vi "Microscope Control.vi"() -> ()   [LabVIEW 2016]
uses:
  Tabs.ctl
panel:
  in  "Stop":bool
  in  "Menu":bool
  in  "MenuCluster":T1
  out "Tab Control":T2
  in  "Access/Refresh Token Path":path
  in  "BMP MAIN FOLDER":path
  in  "Create Page":bool
  in  "Send Image To Onenote?":bool
  out "2D Picture":picture
  out "Current_Inkscape Path":path
  in  "Open_InkScape_dialogue":bool
  # "This will be for all of the settings behind the scenes that the user should not see."
  # "Images"
  # "OneNote"
  # "OneNote Tab"
  # "I should have a control that will let me open the lithography program (this should be done via the command line)."
  # "I wanna show the lithography process as it is happening."
  # "I should get a confirmation that the image is saved and I should also see if I cant display it here."
  # "I think that I want to make a full blown VI that will do literally everything.\nThat means I need to plan out the structure of the VI before I start. I would \nlike to make things like a hamburger menu and a a thing that displays the \ncorrect front panel of whatever im doing etc. In other words I wanna make a boss ass program for the microscope."
  # "The border and label should get hidden."
  # "I should hide the tabs, make this transparent, and then programmatically change the tabs."
  # "Experiment with adding states to the beginning and end of the  queue to change the states a little more  readily..."
  # "ALL NOTES SHOULD GO HERE"
  # "Colors:\nMicroscope: rgb(238,105,66) or near this color\nOnenote:  R128 G57 B123\nPaths: path color (blueish green)\ninkscape"
  # "This  is the Default tab"
  # "The way I shall organize this large undertaking:\nI will make a series of Sub VIs. \nThe main app reference will be in the main VI\nAll references should be opened and closed inside of the sub VIs\nThis will ensure that we will not have any lose hanging references.\nI will also have a series of onenote cases."
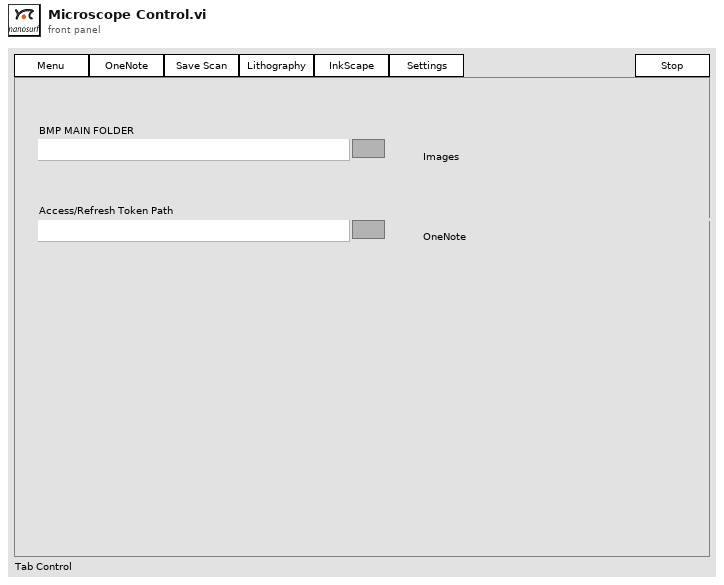
[diagram p1: front panel]
types:
  T1 = cluster{"Settings":bool, "Save Scan":bool, "Perform Lithography":bool, "Open InkScape":bool, "Onenotebutton":bool}
  T2 = typedef "Tabs.ctl" = enum32{"Settings", "Onenote", "Lithography", "Save Image", "InkScape", "Default"}
  T3 = enum32{"invalid app kind", "Development System", "Run Time System", "Student Edition", "Embedded LabVIEW", "Evaluation", "Custom"}
  T4 = enum32{"Invalid", "Standard", "Closed", "Hidden", "Minimized", "Maximized"}
  T5 = cluster{"Core":cluster{"Current VI Reference":refnum<vi>, "Close Panel on Exit?":bool}, "Your Boolean data":bool, "Your string data":string, "Application":refnum<k7>, "Paths":cluster{"BMP_Str":string, "BMP_INK_Str":string, "InkScape_Str":string, "BMP_path":path, "BMP_INK_Path":path, "InkScape_Path":path, "BasePath":path}, "Scan Properties":cluster{"CenterPosX":dbl, "CenterPosY":dbl, "ImageHeight":dbl, "ImageWidth":dbl}, "OneNote":cluster{"Description":string, "Body":cluster{"Description":string, "Path":path}[]}}
  T6 = cluster{"Description":string, "Body":cluster{"Description":string, "Path":path}[]}
  T7 = cluster{"CenterPosX":dbl, "CenterPosY":dbl, "ImageHeight":dbl, "ImageWidth":dbl}
  T8 = cluster{"BMP_Str":string, "BMP_INK_Str":string, "InkScape_Str":string, "BMP_path":path, "BMP_INK_Path":path, "InkScape_Path":path, "BasePath":path}
  T9 = cluster{"Current VI Reference":refnum<vi>, "Close Panel on Exit?":bool}
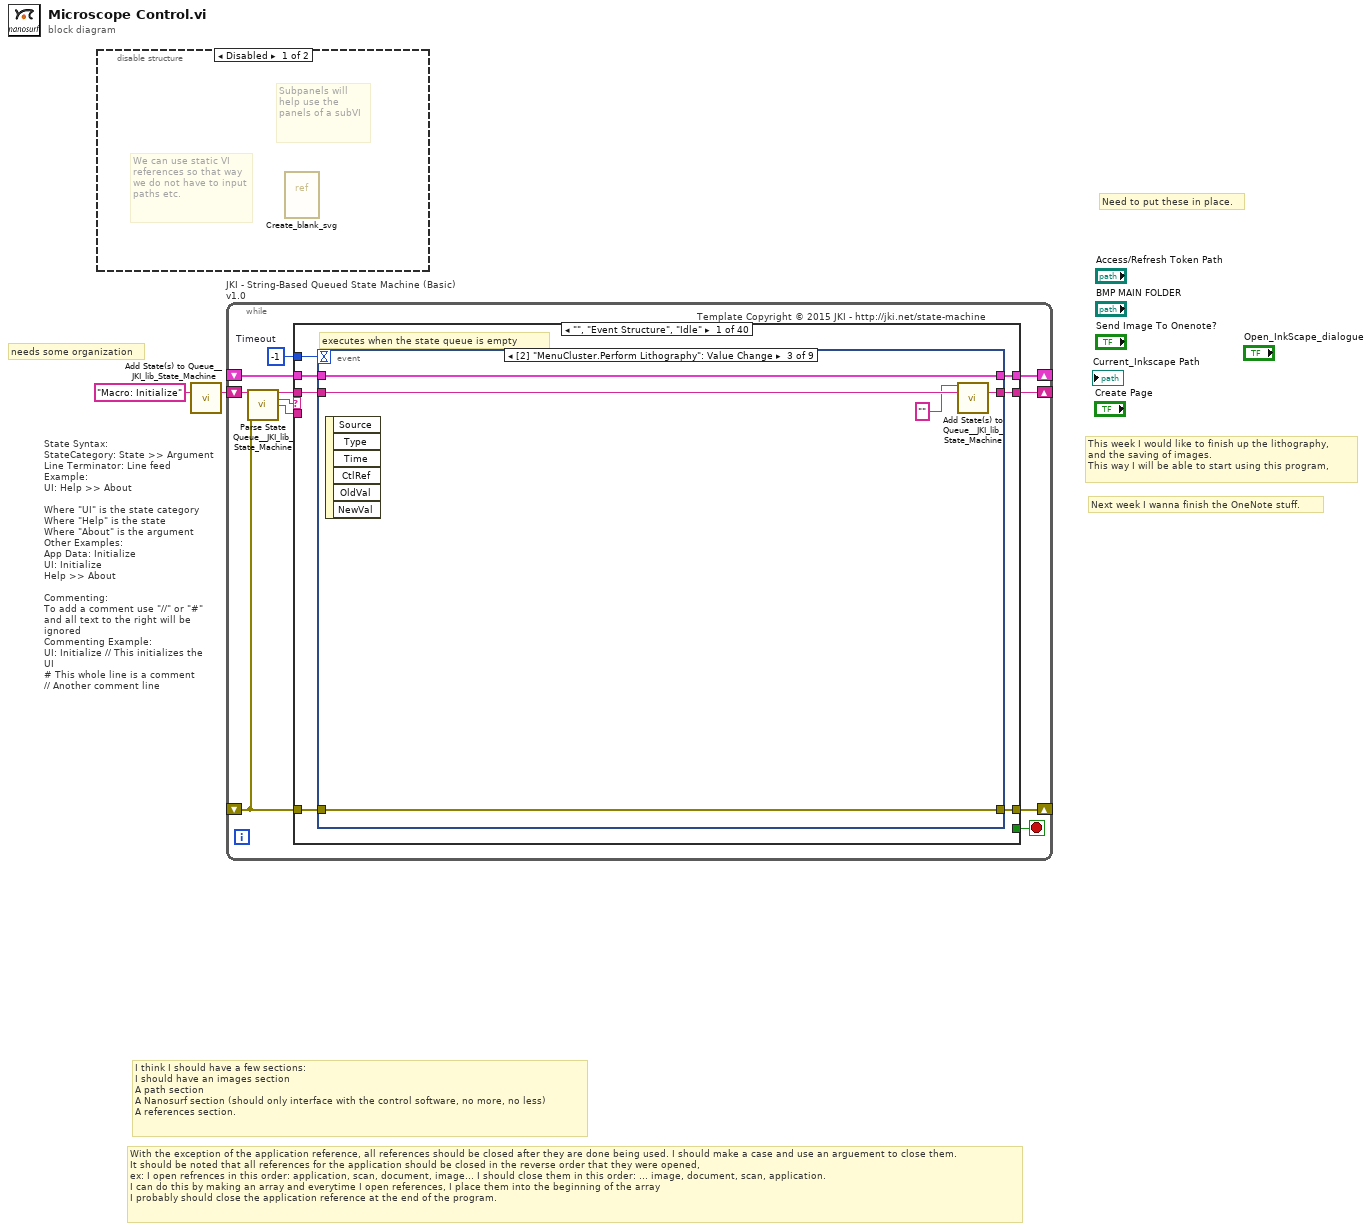
[diagram p0: block diagram]
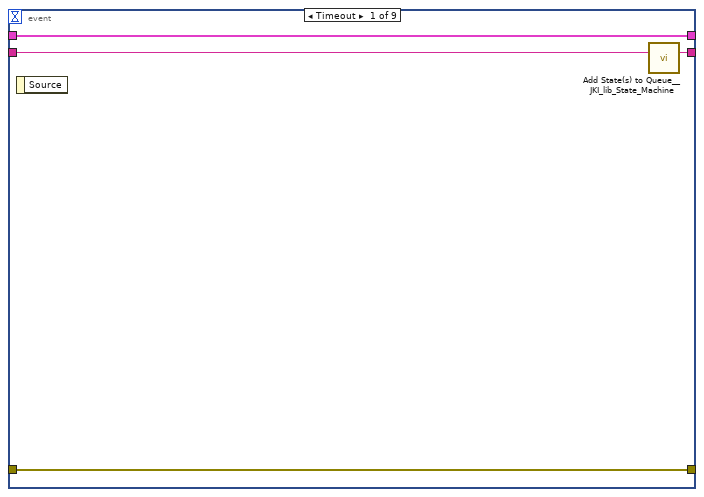
[diagram p3: hidden frame]
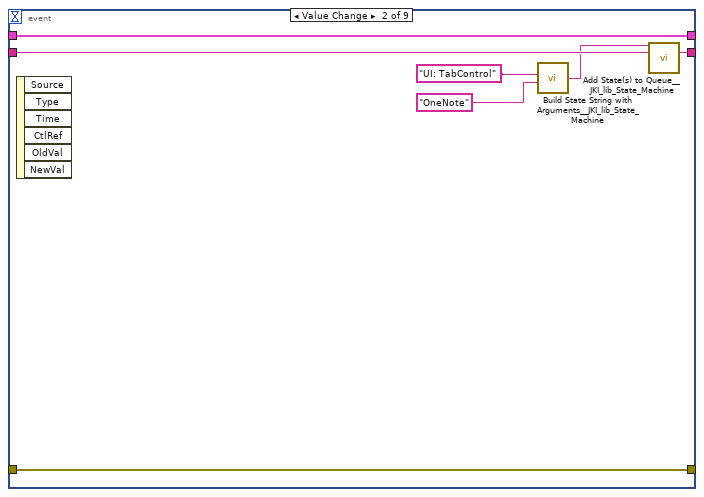
[diagram p4: hidden frame]
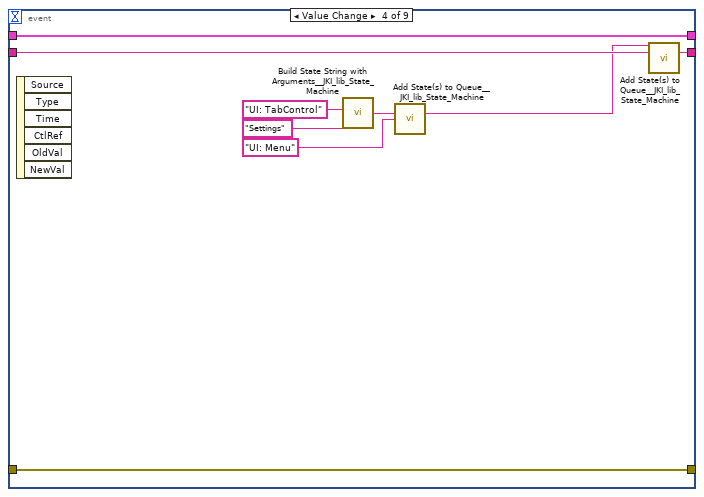
[diagram p5: hidden frame]
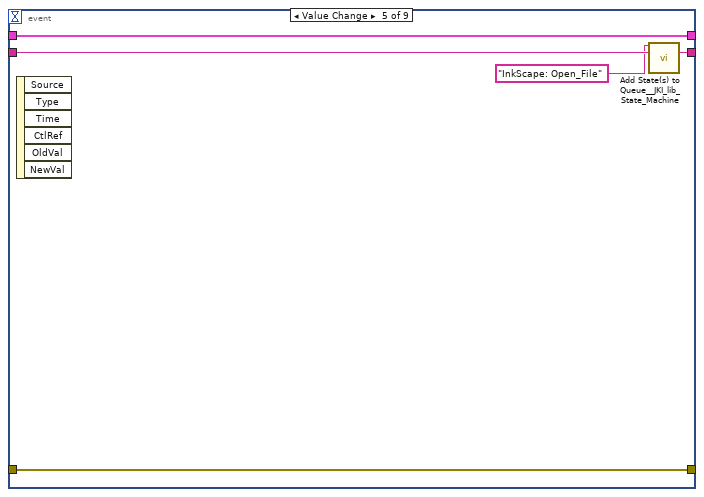
[diagram p6: hidden frame]
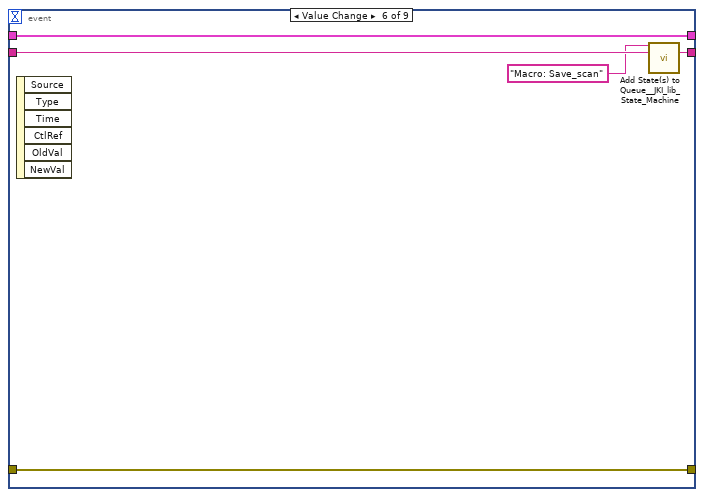
[diagram p7: hidden frame]
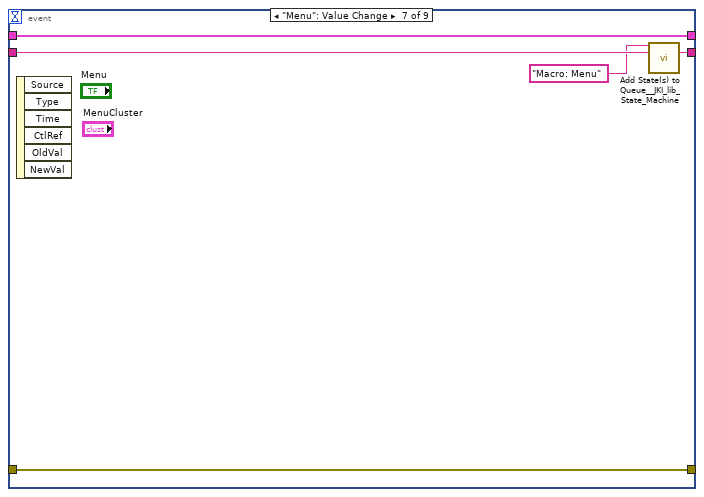
[diagram p8: hidden frame]
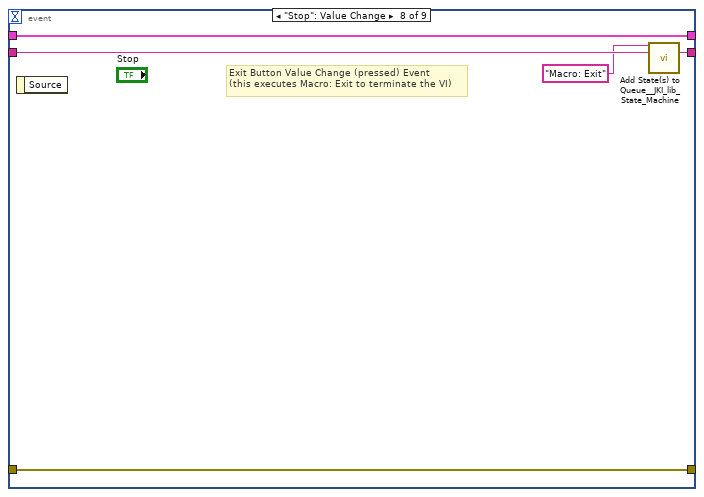
[diagram p9: hidden frame]
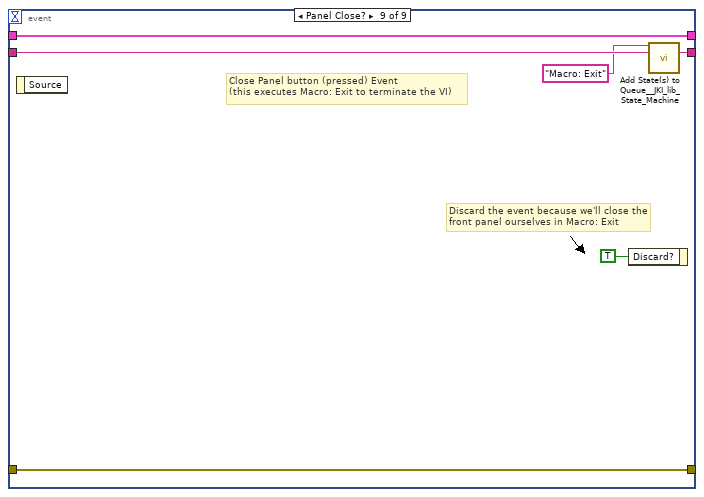
[diagram p10: hidden frame]
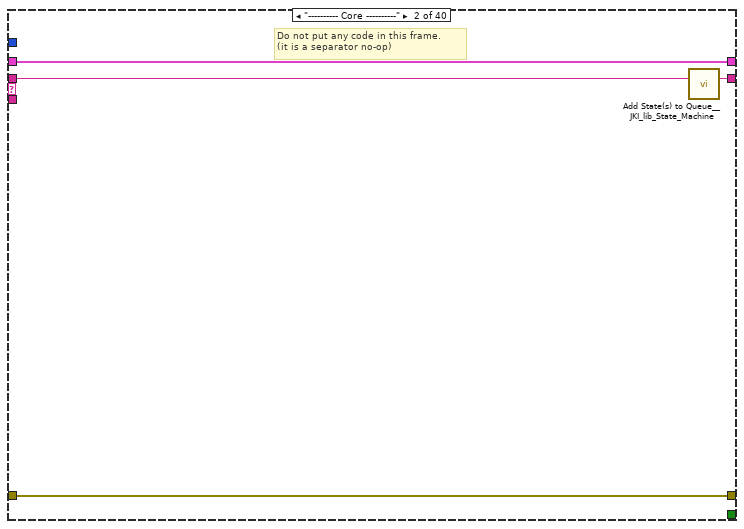
[diagram p11: hidden frame]
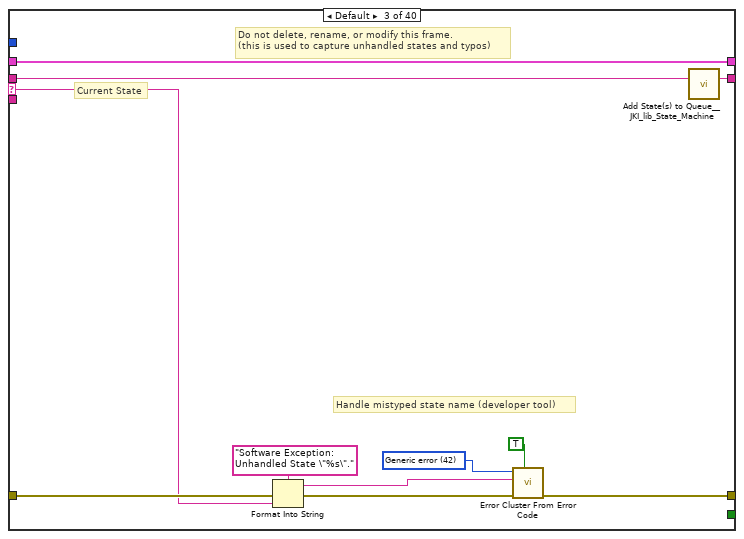
[diagram p12: hidden frame]
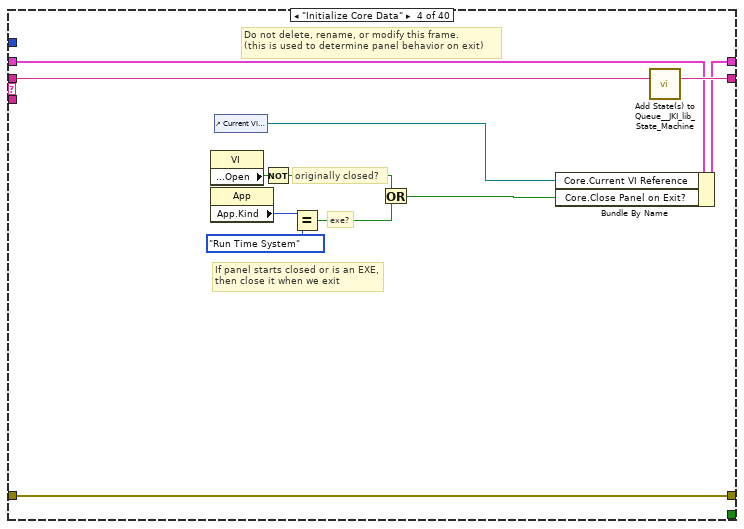
[diagram p13: hidden frame]
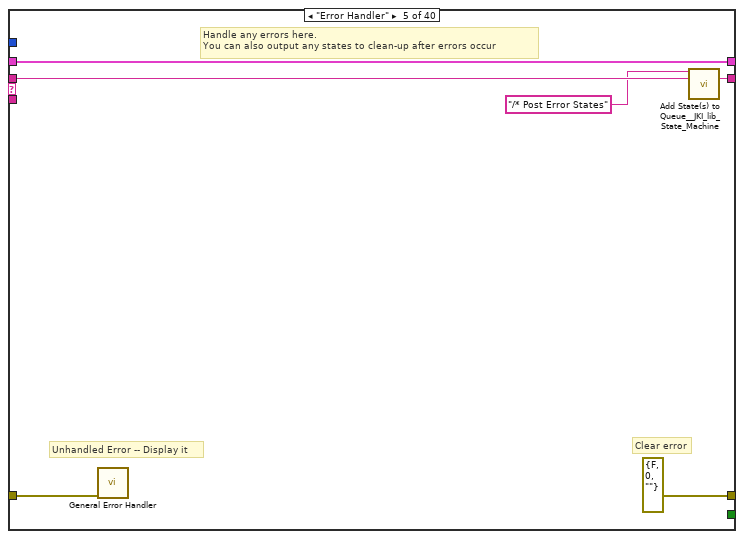
[diagram p14: hidden frame]
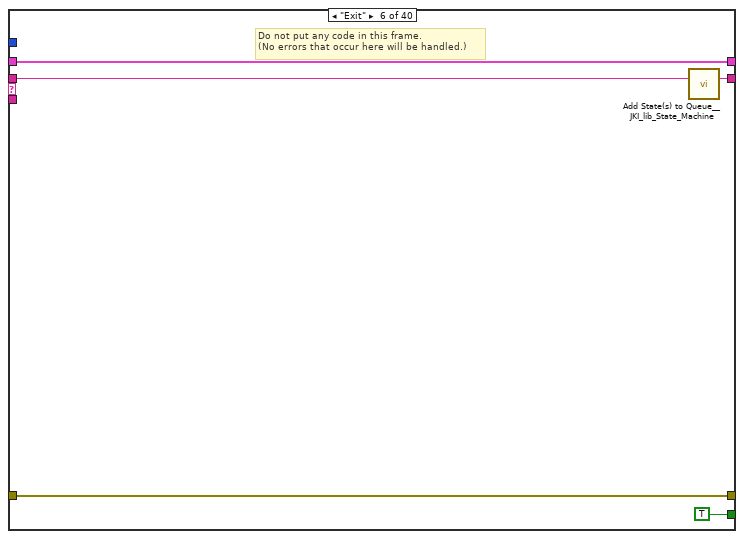
[diagram p15: hidden frame]
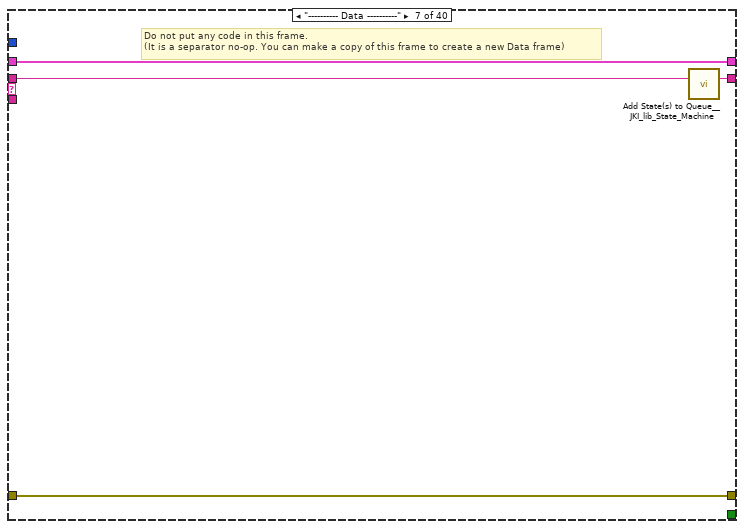
[diagram p16: hidden frame]
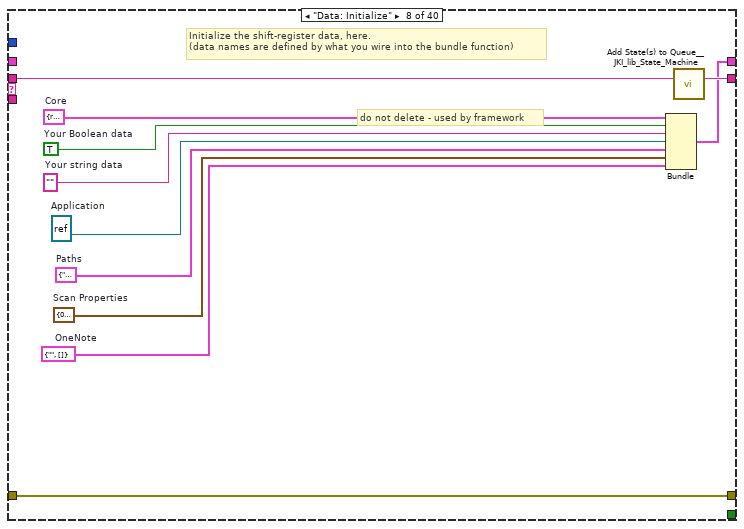
[diagram p17: hidden frame]
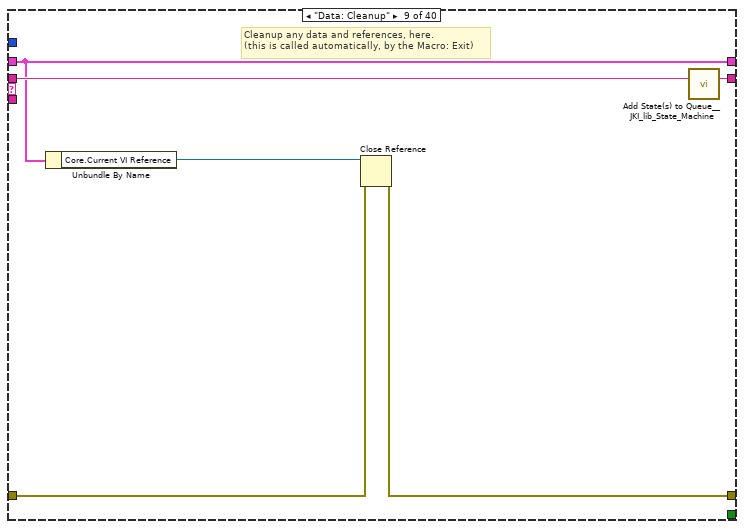
[diagram p18: hidden frame]
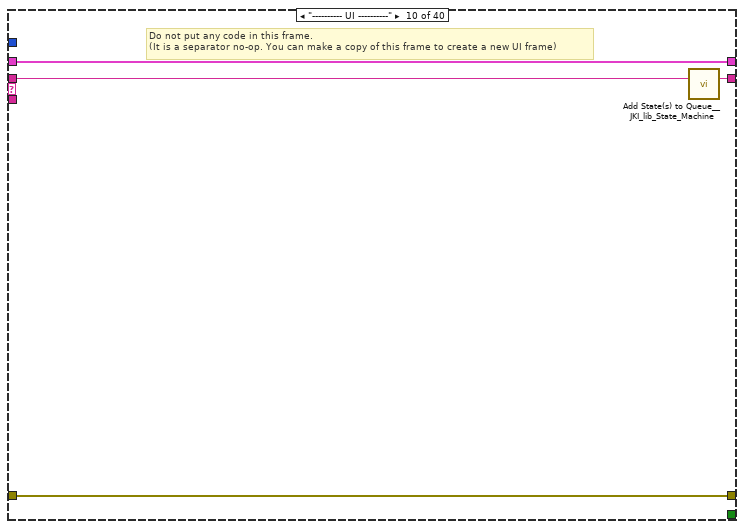
[diagram p19: hidden frame]
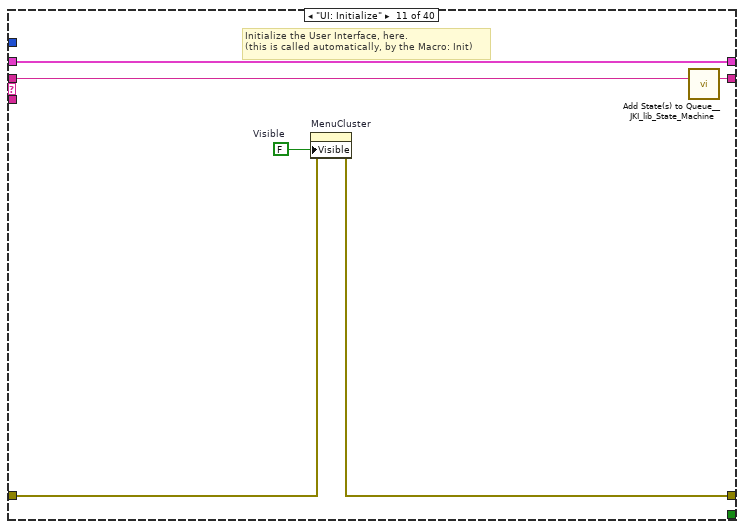
[diagram p20: hidden frame]
diagram:
  # "Need to put these in place."
  # "Next week I wanna finish the OneNote stuff."
  # "This week I would like to finish up the lithography, \nand the saving of images. \nThis way I will be able to start using this program,"
  # "With the exception of the application reference, all references should be closed after they are done being used. I should make a case and use an arguement to close them.\nIt should be noted that all references for the application should be closed in the reverse order that they were opened,\nex: I open refrences in this order: application, scan, document, image... I should close them in this order: ... image, document, scan, application.\nI can do this by making an array and everytime I open references, I place them into the beginning of the array\nI probably should close the application reference at the end of the program."
  # "I think I should have a few sections:\nI should have an images section\nA path section\nA Nanosurf section (should only interface with the control software, no more, no less)\nA references section."
  # "needs some organization"
  # "State Syntax:\nStateCategory: State >> Argument\nLine Terminator: Line feed\nExample:\nUI: Help >> About\n\nWhere \"UI\" is the state category\nWhere \"Help\" is the state\nWhere \"About\" is the argument\nOther Examples:\nApp Data: Initialize\nUI: Initialize\nHelp >> About\n\nCommenting:\nTo add a comment use \"//\" or \"#\" and all text to the right will be ignored\nCommenting Example:\nUI: Initialize // This initializes the UI\n# This whole line is a comment\n// Another comment line"
  n1 = disable-structure shown="Disabled" {
    frame Disabled {
      # "Subpanels will help use the panels of a subVI"
      # "We can use static VI references so that way we do not have to input paths etc."
      n2 = vi-ref "Create_blank_svg.vi"() -> ()  [unwired: 1 out]
    }
    frame Enabled {
    }
  }
  n3 = call <vilib>:"Add State(s) to Queue__JKI_lib_State_Machine.vi"("State(s) in (\"\")"="Macro: Initialize") -> ("States Out"=w2:string)  [unwired: 14 in]
  n4 = while "JKI - String-Based Queued State Machine (Basic) v1.0" {
    shift-right: [w6] -> _
    shift-left: _ -> [w5]
    shift-right: [w9] -> _
    shift-left: _ -> [w3]
    shift-right: [w8] -> _
    shift-left: w2 -> [w10]
    stop <- w7 stop-if-true
    w4 = -1  # Timeout
    # "Template Copyright © 2015 JKI - http://jki.net/state-machine"
    n5 = call <vilib>:"Parse State Queue__JKI_lib_State_Machine.vi"("State Queue"=w10, "Error In (no error)"=w3) -> ("Remaining States"=w12:string, "Current State"=w13:string, "Arguments"=w11:string)  [unwired: 11 in]
    n6 = case shown="\"\", \"Event Structure\", \"Idle\"" w13 {
      selector: w13 -> [_ _ w76 _ _ _ _ _ _ _ _ _ _ _ _ _ _ _ _ _ _ _ _ _ _ _ _ _ _ _ _ _ _ _ _ _ _ _ _ _]
      tunnel: w12 -> [w20 w75 w80 w98 w104 w109 w113 w124 w130 w134 w140 w146 w157 w187 w193 w202 w207 w212 w217 w222 w231 w244 w253 w266 w270 w278 w292 w304 w310 w314 w321 w327 w331 w342 w353 w357 w362 w373 w378 w384]
      tunnel: w11 -> [_ _ _ _ _ _ _ _ _ _ _ w141 w151 _ w188 _ _ _ _ _ _ _ _ _ _ _ _ _ _ _ _ _ _ _ _ _ _ _ _ _]
      tunnel: w5 -> [w18 w72 w78 w89 w101 w107 w110 _ w125 w131 w138 w144 w153 w185 w190 w199 w204 w209 w214 w219 w229 w241 w250 w262 w267 w273 w290 w295 w308 w311 w319 w325 w328 w336 w345 w354 w360 w364 w376 w380]
      tunnel: [w17 w73 w82 w95 errorcluster {"status"=FALSE, "code"=0, "source"=""} ("error out") w106 w111 w121 w126 w132 w135 w142 w154 w180 w191 w200 w205 w210 w215 w220 w227 w242 w251 w263 w268 w275 w280 w302 w305 w312 w315 w322 w329 w339 w346 w355 w358 w371 w374 w381] -> w9
      tunnel: w3 -> [w16 w73 w81 w95 w100 w106 w111 w121 w127 w132 w136 w143 w155 w181 w191 w200 w205 w210 w215 w220 w228 w242 w251 w254 w268 w271 w287 w293 w306 w312 w316 w323 w329 w340 w347 w355 w359 w371 w375 w382]
      tunnel: [w19 w74 w79 w97 w103 w108 w112 w123 w129 w133 w139 w145 w156 w186 w192 w201 w206 w211 w216 w221 w230 w243 w252 w265 w269 w277 w291 w303 w309 w313 w320 w326 w330 w341 w352 w356 w361 w372 w377 w383] -> w8
      tunnel: [_ _ _ _ _ TRUE _ _ _ _ _ _ _ _ _ _ _ _ _ _ _ _ _ _ _ _ _ _ _ _ _ _ _ _ _ _ _ _ _ _] -> w7
      tunnel: [w15 w72 w78 w96 w101 w107 w110 w122 w125 w131 w138 w144 w153 w185 w190 w199 w204 w209 w214 w219 w229 w241 w250 w261 w267 w276 w290 w294 w308 w311 w319 w325 w328 w335 w345 w354 w360 w363 w376 w380] -> w6
      tunnel: w4 -> [w14 _ _ _ _ _ _ _ _ _ _ _ _ _ _ _ _ _ _ _ _ _ _ _ _ _ _ _ _ _ _ _ _ _ _ _ _ _ _ _]
      frame "", "Event Structure", "Idle" {
        # "executes when the state queue is empty"
        n7 = event shown="[2] \"MenuCluster.Perform Lithography\": Value Change" {
          selector: _ -> [_ _ _ _ _ _ _ _ _]
          dyn-events: _ -> [_ _ _ _ _ _ _ _ _]
          timeout: w14 -> [_ _ _ _ _ _ _ _ _]
          tunnel: w20 -> [w24 w31 w36 w45 w50 w55 w60 w65 w71]
          tunnel: [w23 w30 w35 w44 w49 w54 w59 w64 w70] -> w19
          tunnel: w18 -> [w21 w28 w33 w42 w47 w52 w57 w62 w68]
          tunnel: [w22 w29 w34 w43 w48 w53 w58 w63 w69] -> w17
          tunnel: w16 -> [w22 w29 w34 w43 w48 w53 w58 w63 w69]
          tunnel: [w21 w28 w33 w42 w47 w52 w57 w62 w68] -> w15
          event Timeout {
            n8 = event-data() -> ()  [unwired: 1 in, 1 out]
            n9 = call <vilib>:"Add State(s) to Queue__JKI_lib_State_Machine.vi"("State(s) in (\"\")"=w24) -> ("States Out"=w23:string)  [unwired: 14 in]
          }
          event "MenuCluster.Onenotebutton": Value Change {
            n10 = event-data() -> ()  [unwired: 1 in, 6 out]
            n11 = call <vilib>:"Build State String with Arguments__JKI_lib_State_Machine.vi"("Arguments (\"\")"="OneNote" ("Arguments (\"\")"), "State"="UI: TabControl") -> ("State with Arguments"=w26:string)  [unwired: 4 in]
            n12 = call <vilib>:"Add State(s) to Queue__JKI_lib_State_Machine.vi"("State(s) in Front (\"\")"=w26, "State(s) in (\"\")"=w31) -> ("States Out"=w30:string)  [unwired: 13 in]
          }
          event "MenuCluster.Perform Lithography": Value Change {
            n13 = event-data() -> ()  [unwired: 1 in, 6 out]
            n14 = call <vilib>:"Add State(s) to Queue__JKI_lib_State_Machine.vi"("State(s) in Front (\"\")"="" ("State(s) in Front (\"\")"), "State(s) in (\"\")"=w36) -> ("States Out"=w35:string)  [unwired: 13 in]
          }
          event "MenuCluster.Settings": Value Change {
            n15 = event-data() -> ()  [unwired: 1 in, 6 out]
            n16 = call <vilib>:"Build State String with Arguments__JKI_lib_State_Machine.vi"("Arguments (\"\")"="Settings" ("Arguments (\"\")"), "State"="UI: TabControl") -> ("State with Arguments"=w39:string)  [unwired: 4 in]
            n17 = call <vilib>:"Add State(s) to Queue__JKI_lib_State_Machine.vi"("State(s) in (\"\")"=w39, "State(s) at Back (\"\")"="UI: Menu") -> ("States Out"=w37:string)  [unwired: 13 in]
            n18 = call <vilib>:"Add State(s) to Queue__JKI_lib_State_Machine.vi"("State(s) in Front (\"\")"=w37, "State(s) in (\"\")"=w45) -> ("States Out"=w44:string)  [unwired: 13 in]
          }
          event "MenuCluster.Open InkScape": Value Change {
            n19 = event-data() -> ()  [unwired: 1 in, 6 out]
            n20 = call <vilib>:"Add State(s) to Queue__JKI_lib_State_Machine.vi"("State(s) in Front (\"\")"="InkScape: Open_File", "State(s) in (\"\")"=w50) -> ("States Out"=w49:string)  [unwired: 13 in]
          }
          event "MenuCluster.Save Scan": Value Change {
            n21 = event-data() -> ()  [unwired: 1 in, 6 out]
            n22 = call <vilib>:"Add State(s) to Queue__JKI_lib_State_Machine.vi"("State(s) in Front (\"\")"="Macro: Save_scan" ("State(s) in Front (\"\")"), "State(s) in (\"\")"=w55) -> ("States Out"=w54:string)  [unwired: 13 in]
          }
          event "Menu": Value Change {
            n23 = event-data() -> ()  [unwired: 1 in, 6 out]
            n24 = call <vilib>:"Add State(s) to Queue__JKI_lib_State_Machine.vi"("State(s) in Front (\"\")"="Macro: Menu" ("State(s) in Front (\"\")"), "State(s) in (\"\")"=w60) -> ("States Out"=w59:string)  [unwired: 13 in]
          }
          event "Stop": Value Change {
            # "Exit Button Value Change (pressed) Event\n(this executes Macro: Exit to terminate the VI)"
            n25 = event-data() -> ()  [unwired: 1 in, 1 out]
            n26 = call <vilib>:"Add State(s) to Queue__JKI_lib_State_Machine.vi"("State(s) in Front (\"\")"="Macro: Exit", "State(s) in (\"\")"=w65) -> ("States Out"=w64:string)  [unwired: 13 in]
          }
          event Panel Close? {
            # "Discard the event because we'll close the front panel ourselves in Macro: Exit"
            # "Close Panel button (pressed) Event\n(this executes Macro: Exit to terminate the VI)"
            n27 = event-data() -> ()  [unwired: 1 in, 1 out]
            n28 = event-data("Discard?"=TRUE) -> ()  [unwired: 1 in, 1 out]
            n29 = call <vilib>:"Add State(s) to Queue__JKI_lib_State_Machine.vi"("State(s) in Front (\"\")"="Macro: Exit", "State(s) in (\"\")"=w71) -> ("States Out"=w70:string)  [unwired: 13 in]
          }
        }
      }
      frame "---------- Core ----------" {
        # "Do not put any code in this frame.\n(it is a separator no-op)"
        n30 = call <vilib>:"Add State(s) to Queue__JKI_lib_State_Machine.vi"("State(s) in (\"\")"=w75) -> ("States Out"=w74:string)  [unwired: 14 in]
      }
      frame Default {
        w85 = 42 items=["No error", "Argument error", "Memory is full", "Out of zone", "End of file", "File already open", "Generic file I/O error", "File not found", "File permission error", "Disk is full", "Duplicate path", "Too many files open", "System feature not enabled", "Resource file not found", "Cannot add resource", "Resource not found", "Image not found", "Image memory error", "Pen does not exist", "Config type invalid", "Config token not found", "Config parse error", "Config memory error", "Bad external code format", "Bad external code offset", "External code not present", "Null window", "Destroy window error", "Null menu", "Print aborted", "Bad print record", "Print driver error", "Windows error during printing", "Memory error during printing", "Print dialog error", "Generic print error", "Invalid device refnum", "Device not found", "Device parameter error", "Device unit error", "Cannot open device", "Device call aborted", "Generic error", "Cancelled by user", "Object ID too low", "Object ID too high", "Object not in heap", "Unknown heap", "Unknown object (invalid DefProc)", "Unknown object (DefProc not in table)", "Message out of range", "Invalid (null) method", "Unknown message", "Manager call not supported", "Bad address", "Network operation in progress", "Network operation timed out", "Connection is busy", "Network attribute not supported", "Network error", "Address in use", "System out of memory", "Connection aborted", "Connection refused", "Not connected", "Already connected", "Connection closed", "Initialization error (interapplication manager)", "Bad occurrence", "Wait on unbound occurrence handler", "Occurrence queue overflow", "Datalog type conflict", "Unused", "Unrecognized type (interapplication manager)", "Memory corrupt", "Failed to make temporary DLL", "Old CIN version", "Drag socket not found", "Failed to load drop-object", "Failed to register OLE object", "Failed to release OLE object", "Format specifier type mismatch", "Unknown format specifier", "Too few format specifiers", "Too many format specifiers", "Scan failed", "Newer CIN version", "Error converting to variant", "Runtime menu error", "Password tampered", "Variant attribute not found", "Incompatible variant data type", "Event data is not available", "Event Store is not present", "Occurrence is not found", "Event Queue is not created", "Event info is not available", "Refnum passed is NULL", "Error retrieving Class GUID", "Error retrieving CoClass GUID", "Error retrieving TypeLib GUID.", "Bad built application magic bytes.", "Specific driver is different from the specific driver associated with the Logical Name.", "There is no session opened to the class driver.", "Max Error", "MAX - Error with config objects", "MAX - Error loading configuration", "MAX - Group not supported"]
        # "Current State"
        # "Do not delete, rename, or modify this frame.\n(this is used to capture unhandled states and typos)"
        # "Handle mistyped state name (developer tool)"
        n31 = Format Into String(format string="Software Exception: Unhandled State \"%s\"." ("message"), error in=w81, w76) -> (resulting string=w84:string, error out=w83:errorcluster)  [unwired: 1 in]
        n32 = call <vilib>:"Error Cluster From Error Code.vi"("show call chain? (False)"=TRUE, "error in (no error)"=w83, "error message (\"\")"=w84, "error code (0)"=w85) -> ("error out"=w82:errorcluster)  [unwired: 5 in]
        n33 = call <vilib>:"Add State(s) to Queue__JKI_lib_State_Machine.vi"("State(s) in (\"\")"=w80) -> ("States Out"=w79:string)  [unwired: 14 in]
      }
      frame "Initialize Core Data" {
        # "Do not delete, rename, or modify this frame.\n(this is used to determine panel behavior on exit)"
        # "originally closed?"
        # "exe?"
        # "If panel starts closed or is an EXE, then close it when we exit"
        n34 = property class="VI"() -> ("Front Panel.Open"=w94:bool)  [unwired: 2 in, 2 out]
        n35 = property class="App"() -> ("App.Kind"=w93:T3)  [unwired: 2 in, 2 out]
        n36 = control-ref of="Current VI Reference"() -> (w87:refnum<vi>)
        n37 = Not(x=w94) -> (.not. x?=w91:bool)
        n38 = Equal?(x=w93, y=T3."Run Time System" ("Application:Kind")) -> (x = y?=w90:bool)
        n39 = Or(x=w91, y=w90) -> (x .or. y?=w88:bool)
        n40 = Bundle By Name(cluster=w89, "Core.Current VI Reference"=w87, "Core.Close Panel on Exit?"=w88) -> (w96:T5)
        n41 = call <vilib>:"Add State(s) to Queue__JKI_lib_State_Machine.vi"("State(s) in (\"\")"=w98) -> ("States Out"=w97:string)  [unwired: 14 in]
      }
      frame "Error Handler" {
        # "Unhandled Error -- Display it"
        # "Handle any errors here.\nYou can also output any states to clean-up after errors occur"
        # "Clear error"
        n42 = call <vilib>:"General Error Handler.vi"("error in (no error)"=w100) -> ()  [unwired: 10 in, 5 out]
        n43 = call <vilib>:"Add State(s) to Queue__JKI_lib_State_Machine.vi"("State(s) in Front (\"\")"="/* Post Error States", "State(s) in (\"\")"=w104) -> ("States Out"=w103:string)  [unwired: 13 in]
      }
      frame "Exit" {
        # "Do not put any code in this frame.\n(No errors that occur here will be handled.)"
        n44 = call <vilib>:"Add State(s) to Queue__JKI_lib_State_Machine.vi"("State(s) in (\"\")"=w109) -> ("States Out"=w108:string)  [unwired: 14 in]
      }
      frame "---------- Data ----------" {
        # "Do not put any code in this frame.\n(It is a separator no-op. You can make a copy of this frame to create a new Data frame)"
        n45 = call <vilib>:"Add State(s) to Queue__JKI_lib_State_Machine.vi"("State(s) in (\"\")"=w113) -> ("States Out"=w112:string)  [unwired: 14 in]
      }
      frame "Data: Initialize" {
        w114 = T6 {"Description"="", "Body"=[]}  # OneNote
        w115 = T7 {"CenterPosX"=0.0, "CenterPosY"=0.0, "ImageHeight"=0.0, "ImageWidth"=0.0}  # Scan Properties
        w116 = T8 {"BMP_Str"="", "BMP_INK_Str"="", "InkScape_Str"="", "BMP_path"=path "", "BMP_INK_Path"=path "", "InkScape_Path"=path "", "BasePath"=path "C:/Users/monke/Desktop"}  # Paths
        w117 = refnum<k7> refnum  # Application
        w118 = T9 {"Current VI Reference"=refnum, "Close Panel on Exit?"=FALSE}  # Core
        w120 = TRUE  # Your Boolean data
        w119 = ""  # Your string data
        # "do not delete - used by framework"
        # "Initialize the shift-register data, here.\n(data names are defined by what you wire into the bundle function)"
        n46 = Bundle("Core"=w118, "Your Boolean data"=w120, "Your string data"=w119, "Application"=w117, "Paths"=w116, "Scan Properties"=w115, "OneNote"=w114) -> (w122:T5)  [unwired: 1 in]
        n47 = call <vilib>:"Add State(s) to Queue__JKI_lib_State_Machine.vi"("State(s) in (\"\")"=w124) -> ("States Out"=w123:string)  [unwired: 14 in]
      }
      frame "Data: Cleanup" {
        # "Cleanup any data and references, here.\n(this is called automatically, by the Macro: Exit)"
        n48 = Unbundle By Name(w125) -> ("Core.Current VI Reference"=w128:refnum<vi>)
        n49 = Close Reference(reference=w128, error in (no error)=w127) -> (error out=w126:errorcluster)
        n50 = call <vilib>:"Add State(s) to Queue__JKI_lib_State_Machine.vi"("State(s) in (\"\")"=w130) -> ("States Out"=w129:string)  [unwired: 14 in]
      }
      frame "---------- UI ----------" {
        # "Do not put any code in this frame.\n(It is a separator no-op. You can make a copy of this frame to create a new UI frame)"
        n51 = call <vilib>:"Add State(s) to Queue__JKI_lib_State_Machine.vi"("State(s) in (\"\")"=w134) -> ("States Out"=w133:string)  [unwired: 14 in]
      }
      frame "UI: Initialize" {
        w137 = FALSE  # Visible
        # "Initialize the User Interface, here.\n(this is called automatically, by the Macro: Init)"
        n52 = property on="MenuCluster" class="Clust"(error in=w136, "Visible"=w137) -> (error out=w135:errorcluster)  [unwired: 1 in, 1 out]
        n53 = call <vilib>:"Add State(s) to Queue__JKI_lib_State_Machine.vi"("State(s) in (\"\")"=w140) -> ("States Out"=w139:string)  [unwired: 14 in]
      }
      frame "UI: Cursor Set" {
        # "Argument"
        # "Set and Unset Cursor Busy.\n(Usage: \"UI: Cursor Set >> Busy|Idle\")"
        n54 = case shown="\"Idle\", Default" w141 {
          tunnel: w143 -> [w148 w150]
          tunnel: [w147 w149] -> w142
          frame "Idle", Default {
            n55 = call <vilib>:"Unset Busy.vi"("error in (no error)"=w148) -> ("error out"=w147:errorcluster)  [unwired: 10 in]
          }
          frame "Busy" {
            n56 = call <vilib>:"Set Busy.vi"("error in (no error)"=w150) -> ("error out"=w149:errorcluster)  [unwired: 9 in, 1 out]
          }
        }
        n57 = call <vilib>:"Add State(s) to Queue__JKI_lib_State_Machine.vi"("State(s) in (\"\")"=w146) -> ("States Out"=w145:string)  [unwired: 14 in]
      }
      frame "UI: Front Panel State" {
        # "Argument"
        # "Set Front Panel Open or Closed\n(Usage: \"UI: Front Panel State >> Open|Close\")"
        n58 = Unbundle By Name(w153) -> ("Core.Current VI Reference"=w152:refnum<vi>)
        n59 = case shown="\"Open\", Default" w151 {
          tunnel: w155 -> [w161 w174]
          tunnel: [w163 w175] -> w154
          tunnel: w152 -> [w162 w172]
          frame "Open", Default {
            n60 = property class="VI"(reference=w162, error in=w161) -> (reference out=w159:refnum<vi>, error out=w160:errorcluster, "Front Panel.Open"=w158:bool)
            n61 = case shown="False" w158 {
              tunnel: [w166 w169] -> w163
              tunnel: w160 -> [w165 w169]
              tunnel: w159 -> [w164 _]
              frame False {
                n62 = invoke class="VI" method="FP.Open"(reference=w164, error in=w165, "Activate"=TRUE, "State"=T4."Standard") -> (error out=w166:errorcluster)  [unwired: 1 in, 4 out]
              }
              frame True {
              }
            }
          }
          frame "Close" {
            n63 = property class="VI"(reference=w172, error in=w174) -> (reference out=w171:refnum<vi>, error out=w173:errorcluster, "Front Panel.Open"=w170:bool)
            n64 = case shown="True" w170 {
              tunnel: [w176 w179] -> w175
              tunnel: w173 -> [w176 w178]
              tunnel: w171 -> [_ w177]
              frame False {
              }
              frame True {
                n65 = invoke class="VI" method="FP.Close"(reference=w177, error in=w178) -> (error out=w179:errorcluster)  [unwired: 1 in, 2 out]
              }
            }
          }
        }
        n66 = call <vilib>:"Add State(s) to Queue__JKI_lib_State_Machine.vi"("State(s) in (\"\")"=w157) -> ("States Out"=w156:string)  [unwired: 14 in]
      }
      frame "UI: Menu" {
        # "Do not put any code in this frame.\n(It is a separator no-op. You can make a copy of this frame to create a new UI frame)"
        n67 = property on="MenuCluster" class="Clust"(error in=w181) -> (error out=w182:errorcluster, "Visible"=w184:bool)  [unwired: 1 in, 1 out]
        n68 = Not(x=w184) -> (.not. x?=w183:bool)
        n69 = property on="MenuCluster" class="Clust"(error in=w182, "Visible"=w183) -> (error out=w180:errorcluster)  [unwired: 1 in, 1 out]
        n70 = call <vilib>:"Add State(s) to Queue__JKI_lib_State_Machine.vi"("State(s) in (\"\")"=w187) -> ("States Out"=w186:string)  [unwired: 14 in]
      }
      frame "UI: TabControl" {
        n71 = case shown="\"OneNote\"" w188 {
          tunnel: [w194 w195 w196 w197 w198] -> w189
          frame "Normal", Default {
            w194 = Tabs."Default"  # Tab Control
          }
          frame "OneNote" {
            w195 = Tabs."Onenote"  # Tab Control
          }
          frame "Save" {
            w196 = Tabs."Default"  # Tab Control
          }
          frame "Lithography" {
            w197 = Tabs."Lithography"  # Tab Control
          }
          frame "Settings" {
            w198 = Tabs."Settings"  # Tab Control
          }
        }
        "Tab Control" <- w189
        n72 = call <vilib>:"Add State(s) to Queue__JKI_lib_State_Machine.vi"("State(s) in (\"\")"=w193) -> ("States Out"=w192:string)  [unwired: 14 in]
      }
      frame "---------- Macro ----------" {
        # "Do not put any code in this frame.\n(It is a separator no-op. You can make a copy of this frame to create a new Macro frame)"
        n73 = call <vilib>:"Add State(s) to Queue__JKI_lib_State_Machine.vi"("State(s) in (\"\")"=w202) -> ("States Out"=w201:string)  [unwired: 14 in]
      }
      frame "Macro: Initialize" {
        w203 = "Data: Initialize\nInitialize Core Data\nUI: Initialize\nUI: Front Panel State >> Open\nUI: TabControl>>Normal\n//Nanosurf: start application"  # Data: Initialize Initialize Core Data UI: Initialize UI: Front Panel State >> Open UI: TabControl>>Normal //Nanosurf: start application
        # "Initialization Macro\n(This is called once, when the VI starts)"
        n74 = call <vilib>:"Add State(s) to Queue__JKI_lib_State_Machine.vi"("State(s) in Front (\"\")"=w203, "State(s) in (\"\")"=w207) -> ("States Out"=w206:string)  [unwired: 13 in]
      }
      frame "Macro: Menu" {
        # "Do not put any code in this frame.\n(It is a separator no-op. You can make a copy of this frame to create a new Macro frame)"
        n75 = call <vilib>:"Add State(s) to Queue__JKI_lib_State_Machine.vi"("State(s) in Front (\"\")"="UI: Menu" ("State(s) in Front (\"\")"), "State(s) in (\"\")"=w212) -> ("States Out"=w211:string)  [unwired: 13 in]
      }
      frame "Macro: Settings" {
        # "Do not put any code in this frame.\n(It is a separator no-op. You can make a copy of this frame to create a new Macro frame)"
        n76 = call <vilib>:"Add State(s) to Queue__JKI_lib_State_Machine.vi"("State(s) in Front (\"\")"="UI: TabControl>> Settings\nUI: Menu", "State(s) in (\"\")"=w217) -> ("States Out"=w216:string)  [unwired: 13 in]
      }
      frame "Macro: Save_scan" {
        (unwired) "Paths: New\nNanosurf: save BMP\nNanosurf: Scan Properties\nImages: copy_bmp_for_inkscape\nImages: BMP_INK_Properties\nInkScape: Create_New"
        # "This is the correct one."
        # "Get file paths\nSave scan as a BMP\nMake a copy of BMP\nMake an SVG file with the image already linked\nmake an NID file \nclose the NID file.\nOpen up the inkscape file."
        # "Do not put any code in this frame.\n(It is a separator no-op. You can make a copy of this frame to create a new Macro frame)"
        n77 = call <vilib>:"Add State(s) to Queue__JKI_lib_State_Machine.vi"("State(s) in Front (\"\")"="", "State(s) in (\"\")"=w222) -> ("States Out"=w221:string)  [unwired: 13 in]
      }
      frame "Macro: Cloud" {
        w223 = ""  # Connected
        w225 = ""  # Not Connected
        # "To check timeout:\nGet auth in the beginning and also the current time.\nThen set a time for the expiration to be 3300s into the future (55 minutes into the future)\nEvery time you do a request, check the time against this set time.\n->If greater than or equal to refresh\n->if less than make a request using the stuff that you have."
        # "Check if connected to the internet"
        n78 = call "Check_connection.vi"("error in (no error)"=w228) -> ("Internet Connected?"=w226:bool, "error out"=w227:errorcluster)  [unwired: 8 in]
        n79 = Select(t=w223, s=w226, f=w225) -> (s? t:f=w224:string)
        n80 = call <vilib>:"Add State(s) to Queue__JKI_lib_State_Machine.vi"("State(s) in Front (\"\")"=w224, "State(s) in (\"\")"=w231) -> ("States Out"=w230:string)  [unwired: 13 in]
      }
      frame "Macro: Exit" {
        w232 = TRUE  # In Developement?
        # "Exit Macro\n(This is called once, when the VI exits)"
        n81 = Unbundle By Name(w241) -> ("Core.Close Panel on Exit?"=w240:bool)
        n82 = case shown="True" w232 {
          tunnel: [w248 "" ("f")] -> w233
          frame False {
            n83 = property on="MenuCluster" class="Clust"() -> ("Visible"=w247:bool)  [unwired: 2 in, 2 out]
            n84 = Select(t="UI: Menu", s=w247, f="") -> (s? t:f=w248:string)
          }
          frame True {
          }
        }
        n85 = call <vilib>:"Add State(s) to Queue__JKI_lib_State_Machine.vi"("State(s) in (\"\")"=w233, "State(s) at Back (\"\")"="//Nanosurf: Close Application\nData: Cleanup\nExit") -> ("States Out"=w234:string)  [unwired: 13 in]
        n86 = Select(t="UI: Front Panel State >> Close", s=w240, f="") -> (s? t:f=w237:string)
        n87 = call <vilib>:"Add State(s) to Queue__JKI_lib_State_Machine.vi"("State(s) in (\"\")"=w237, "State(s) at Back (\"\")"=w234) -> ("States Out"=w236:string)  [unwired: 13 in]
        n88 = call <vilib>:"Add State(s) to Queue__JKI_lib_State_Machine.vi"("State(s) in Front (\"\")"=w236, "State(s) in (\"\")"=w244) -> ("States Out"=w243:string)  [unwired: 13 in]
      }
      frame "---------- Paths ----------" {
        # "Do not put any code in this frame.\n(It is a separator no-op. You can make a copy of this frame to create a new Macro frame)"
        n89 = call <vilib>:"Add State(s) to Queue__JKI_lib_State_Machine.vi"("State(s) in (\"\")"=w253) -> ("States Out"=w252:string)  [unwired: 14 in]
      }
      frame "Paths: New" {
        # "Do not put any code in this frame.\n(It is a separator no-op. You can make a copy of this frame to create a new Macro frame)"
        n90 = Unbundle By Name(w262) -> ("Paths.BasePath"=w264:path)
        n91 = call "Generic file paths.vi"("error in (no error)"=w254, "Parent Folder"=w264) -> ("error out"=w263:errorcluster, "SVG Path"=w255:string, "BMP for inkscape path"=w256:string, "BMP Path"=w260:string)  [unwired: 6 in]
        n92 = String To Path(string=w260) -> (path=w259:path)
        n93 = String To Path(string=w256) -> (path=w258:path)
        n94 = String To Path(string=w255) -> (path=w257:path)
        n95 = Bundle By Name(cluster=w262, "Paths.BMP_Str"=w260, "Paths.BMP_path"=w259, "Paths.BMP_INK_Str"=w256, "Paths.BMP_INK_Path"=w258, "Paths.InkScape_Str"=w255, "Paths.InkScape_Path"=w257) -> (w261:T5)
        n96 = call <vilib>:"Add State(s) to Queue__JKI_lib_State_Machine.vi"("State(s) in (\"\")"=w266) -> ("States Out"=w265:string)  [unwired: 14 in]
      }
      frame "---------- Nanosurf ----------" {
        # "Do not put any code in this frame.\n(It is a separator no-op. You can make a copy of this frame to create a new Macro frame)"
        n97 = call <vilib>:"Add State(s) to Queue__JKI_lib_State_Machine.vi"("State(s) in (\"\")"=w270) -> ("States Out"=w269:string)  [unwired: 14 in]
      }
      frame "Nanosurf: start application" {
        n98 = Unbundle By Name(w273) -> ("Application"=w272:refnum<k7>)
        n99 = Automation Open(error in (no error)=w271, Automation Refnum=w272) -> (Automation Refnum=w274:refnum<k7>, error out=w275:errorcluster)  [unwired: 2 in]
        n100 = Bundle By Name(cluster=w273, "Application"=w274) -> (w276:T5)
        n101 = call <vilib>:"Add State(s) to Queue__JKI_lib_State_Machine.vi"("State(s) in (\"\")"=w278) -> ("States Out"=w277:string)  [unwired: 14 in]
      }
      frame "Nanosurf: save BMP" {
        w279 = i16 500  # Max Width
        # "Need to add all of the fancy stuff for sizing but this should do for now."
        n102 = Unbundle By Name(w290) -> ("Paths.BMP_path"=w289:path, "Application"=w288:refnum<k7>)
        n103 = call "Save_scan_as_BMP_sub_vi.vi"("error in (no error)"=w287, "Application"=w288, "BMP Path In"=w289) -> ("Error Out"=w281:errorcluster, "BMP"=→"2D Picture":picture, "BMP Path Out"=w285:path)  [unwired: 6 in]
        n104 = control-ref of="2D Picture"() -> (w286:refnum<vi>)
        n105 = call <userlib>:"Draw Image from File__ogtk.vi"("error in (no error)"=w281, "path to image file"=w285) -> ("error out"=w282:errorcluster, "image size (pixels)"=w284:cluster{"x":i16, "y":i16})  [unwired: 6 in, 2 out]
        n106 = call "onenote_dialog_Fit_image_max_size.vi"("error in (no error)"=w282, "Max Width"=w279, "image size (pixels)"=w284, "Picture Refnum"=w286) -> ("error out"=w280:errorcluster)  [unwired: 7 in]
        n107 = call <vilib>:"Add State(s) to Queue__JKI_lib_State_Machine.vi"("State(s) in (\"\")"=w292) -> ("States Out"=w291:string)  [unwired: 14 in]
      }
      frame "Nanosurf: Scan Properties" {
        n108 = Unbundle By Name(w295) -> ("Application"=w301:refnum<k7>)
        n109 = call "Scan Properties.vi"("error in (no error)"=w293, "Application"=w301) -> ("error out"=w302:errorcluster, "Scan Properties"=w300:T7)  [unwired: 8 in]
        n110 = Unbundle(w300) -> ("CenterPosX"=w299:dbl, "CenterPosY"=w298:dbl, "ImageHeight"=w297:dbl, "ImageWidth"=w296:dbl)
        n111 = Bundle By Name(cluster=w295, "Scan Properties.CenterPosX"=w299, "Scan Properties.CenterPosY"=w298, "Scan Properties.ImageHeight"=w297, "Scan Properties.ImageWidth"=w296) -> (w294:T5)
        n112 = call <vilib>:"Add State(s) to Queue__JKI_lib_State_Machine.vi"("State(s) in (\"\")"=w304) -> ("States Out"=w303:string)  [unwired: 14 in]
      }
      frame "Nanosurf: Close Application" {
        # "Do not put any code in this frame.\n(It is a separator no-op. You can make a copy of this frame to create a new Macro frame)"
        n113 = Unbundle By Name(w308) -> ("Application"=w307:refnum<k7>)
        n114 = Close Reference(reference=w307, error in (no error)=w306) -> (error out=w305:errorcluster)
        n115 = call <vilib>:"Add State(s) to Queue__JKI_lib_State_Machine.vi"("State(s) in (\"\")"=w310) -> ("States Out"=w309:string)  [unwired: 14 in]
      }
      frame "---------- Images ----------" {
        # "Do not put any code in this frame.\n(It is a separator no-op. You can make a copy of this frame to create a new Macro frame)"
        n116 = call <vilib>:"Add State(s) to Queue__JKI_lib_State_Machine.vi"("State(s) in (\"\")"=w314) -> ("States Out"=w313:string)  [unwired: 14 in]
      }
      frame "Images: copy_bmp_for_inkscape" {
        n117 = Unbundle By Name(w319) -> ("Paths.BMP_path"=w318:path, "Paths.BMP_INK_Path"=w317:path)
        n118 = Copy(8:w316, 10:w317, 11:w318) -> (0:w315:errorcluster)  [unwired: 2 in, 2 out]
        n119 = call <vilib>:"Add State(s) to Queue__JKI_lib_State_Machine.vi"("State(s) in (\"\")"=w321) -> ("States Out"=w320:string)  [unwired: 14 in]
      }
      frame "Images: BMP_INK_Properties" {
        n120 = Unbundle By Name(w325) -> ("Paths.BMP_INK_Path"=w324:path)
        n121 = call "Change_image_properties.vi"("error in (no error)"=w323, "Path In"=w324) -> ("error out"=w322:errorcluster)  [unwired: 8 in, 1 out]
        n122 = call <vilib>:"Add State(s) to Queue__JKI_lib_State_Machine.vi"("State(s) in (\"\")"=w327) -> ("States Out"=w326:string)  [unwired: 14 in]
      }
      frame "---------- InkScape ----------" {
        # "Do not put any code in this frame.\n(It is a separator no-op. You can make a copy of this frame to create a new Macro frame)"
        n123 = call <vilib>:"Add State(s) to Queue__JKI_lib_State_Machine.vi"("State(s) in (\"\")"=w331) -> ("States Out"=w330:string)  [unwired: 14 in]
      }
      frame "InkScape: Create_New" {
        n124 = Unbundle By Name(w336) -> ("Paths.InkScape_Str"=w338:string, "Paths.BMP_INK_Str"=w337:string, "Scan Properties.ImageHeight"=w333:dbl, "Scan Properties.ImageWidth"=w332:dbl)
        n125 = call "Create_blank_svg.vi"("SVG Path"=w338, "BMP for inkscape path"=w337, "HEIGHT"=w333, "WIDTH"=w332, "error in"=w340) -> ("SVG Path Out"=w334:path, "error out"=w339:errorcluster)  [unwired: 9 in]
        n126 = Bundle By Name(cluster=w336, "Paths.InkScape_Path"=w334) -> (w335:T5)
        n127 = call <vilib>:"Add State(s) to Queue__JKI_lib_State_Machine.vi"("State(s) in (\"\")"=w342) -> ("States Out"=w341:string)  [unwired: 14 in]
      }
      frame "InkScape: Open_File" {
        w343 = FALSE  # wait until completion?
        w348 = TRUE  # run minimized?
        w350 = "\""  # string
        w351 = "cmd /c \""  # string
        # "Do not put any code in this frame.\n(It is a separator no-op. You can make a copy of this frame to create a new Macro frame)"
        n128 = Unbundle By Name(w345) -> ("Paths.InkScape_Str"=w344:string)
        n129 = Concatenate Strings(w351, w344, w350) -> (w349:string)
        n130 = call <vilib>:"System Exec.vi"("run minimized? (F)"=w348, "wait until completion? (T)"=w343, "error in (no error)"=w347, "command line"=w349) -> ("error out"=w346:errorcluster)  [unwired: 4 in, 3 out]
        n131 = call <vilib>:"Add State(s) to Queue__JKI_lib_State_Machine.vi"("State(s) in (\"\")"=w353) -> ("States Out"=w352:string)  [unwired: 14 in]
      }
      frame "---------- OneNote ----------" {
        # "Do not put any code in this frame.\n(It is a separator no-op. You can make a copy of this frame to create a new Macro frame)"
        n132 = call <vilib>:"Add State(s) to Queue__JKI_lib_State_Machine.vi"("State(s) in (\"\")"=w357) -> ("States Out"=w356:string)  [unwired: 14 in]
      }
      frame "OneNote: Auth" {
        # "Need to place into data a path for codes,\nAuthentificaition timer."
        n133 = call "Onenote_Auth_handler.vi"("error in (no error)"=w359) -> ("error out"=w358:errorcluster)  [unwired: 8 in, 2 out]
        n134 = call <vilib>:"Add State(s) to Queue__JKI_lib_State_Machine.vi"("State(s) in (\"\")"=w362) -> ("States Out"=w361:string)  [unwired: 14 in]
      }
      frame "OneNote: Add Picture" {
        # "Do not put any code in this frame.\n(It is a separator no-op. You can make a copy of this frame to create a new Macro frame)"
        n135 = Unbundle By Name(w364) -> ("OneNote.Body"=w368:cluster{"Description":string, "Path":path}[], "OneNote.Description"=w367:string, "Paths.BMP_path"=w366:path)
        n136 = Bundle(cluster=cluster{"Description":string, "Path":path} {"Description"="", "Path"=path ""} ("Cluster"), "Description"=w367, "Path"=w366) -> (w370:cluster{"Description":string, "Path":path})
        n137 = Build Array (concatenate)(w368, w370) -> (w365:cluster{"Description":string, "Path":path}[])
        n138 = Bundle By Name(cluster=w364, "OneNote.Body"=w365) -> (w363:T5)
        n139 = call <vilib>:"Add State(s) to Queue__JKI_lib_State_Machine.vi"("State(s) in (\"\")"=w373) -> ("States Out"=w372:string)  [unwired: 14 in]
      }
      frame "OneNote: Page_Content" {
        # "This VI will help one format their request. It  should pop up and allow the user to format their data. Also it should have sensible resizing of the front panel and all of the objects. This will take up a large part of the work."
        n140 = call "onenote_dialogue.vi"("error in (no error)"=w375) -> ("error out"=w374:errorcluster)  [unwired: 8 in, 2 out]
        n141 = call <vilib>:"Add State(s) to Queue__JKI_lib_State_Machine.vi"("State(s) in (\"\")"=w378) -> ("States Out"=w377:string)  [unwired: 14 in]
      }
      frame "OneNote: Send" {
        # "Do not put any code in this frame.\n(It is a separator no-op. You can make a copy of this frame to create a new Macro frame)"
        n142 = Unbundle By Name(w380) -> ("OneNote.Body"=w379:cluster{"Description":string, "Path":path}[])
        n143 = disable-structure shown="Disabled" {
          disable-tunnel: w382 -> [w387 _]
          disable-tunnel: [w386 _] -> w381
          disable-tunnel: w379 -> [w385 _]
          frame Disabled {
            n144 = call "Send_to_ONENOTE.vi"("Error In"=w387, "Body"=w385) -> ("Error Out"=w386:errorcluster)  [unwired: 7 in, 2 out]
          }
          frame Enabled {
          }
        }
        n145 = call <vilib>:"Add State(s) to Queue__JKI_lib_State_Machine.vi"("State(s) in (\"\")"=w384) -> ("States Out"=w383:string)  [unwired: 14 in]
      }
    }
  }
